vi "get All Data.vi"(0 "identifier":string, 1 "Board":u16, 2 "values":u16, 3 "id":u32, 4 "stats":dbl, 5 "advstats":cluster{}, 6 "spectra_size":u32, 7 "error in (no error)":errorcluster, 8 "data_number":u32) -> (18 "data_number out":u32, 20 "function return":bool, 22 "values out":u16, 23 "id out":u32, 24 "stats out":dbl, 25 "advstats out":cluster{}, 26 "spectra_size out":u32, 27 "error out":errorcluster)   [LabVIEW 2015, in "XGL_DPP.lvlib"]
doc: "EXTERN DECLSPEC bool CALL_CONV getAllData(const char * identifier,\n uint16_t Board,\n uint16_t * values,\n uint32_t * id,\n double* stats,\n uint64_t * advstats,\n uint32_t * spectra_size,\n uint32_t * data_number\n);"
uses:
  XGL_DPP.lvlib
  XGL_DPP.dll
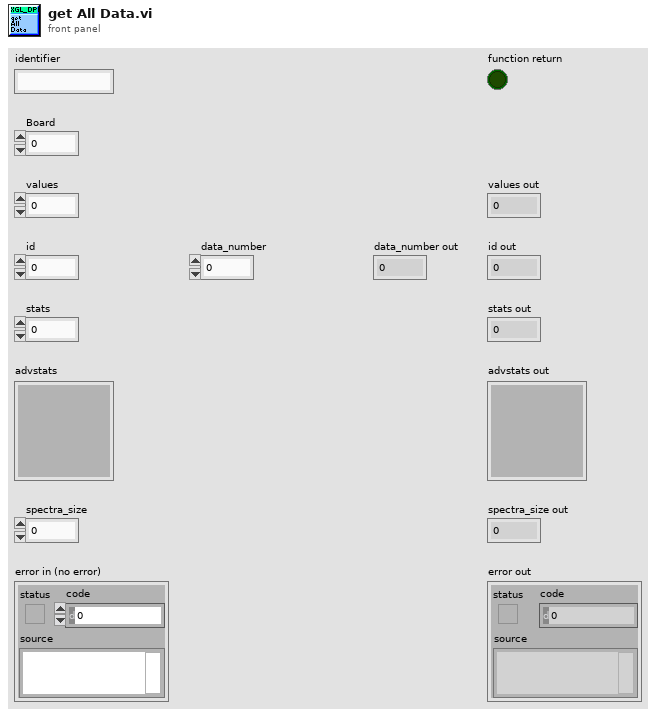
[diagram p1: front panel]
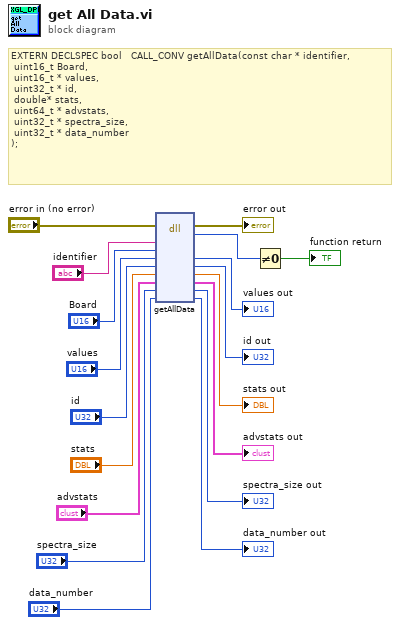
[diagram p0: block diagram]
diagram:
  # "EXTERN DECLSPEC bool   CALL_CONV getAllData(const char * identifier,\n\tuint16_t Board,\n\tuint16_t * values,\n\tuint32_t * id,\n\tdouble* stats,\n\tuint64_t * advstats,\n\tuint32_t * spectra_size,\n\tuint32_t * data_number\n);"
  n1 = dll-call lib="D:/Users/XRF/Desktop/Scanning Software_Demokritos_2015_v7/libs/Vis_2/XGL_DPP.*" fn="getAllData"(error in="error in (no error)", "identifier"="identifier", "Board"="Board", "values"="values", "id"="id", "stats"="stats", "advstats"="advstats", "spectra_size"="spectra_size", "data_number"="data_number") -> (error out=→"error out":errorcluster, w17:u8, "values"=→"values out":u16, "id"=→"id out":u32, "stats"=→"stats out":dbl, "advstats"=→"advstats out":cluster{}, "spectra_size"=→"spectra_size out":u32, "data_number"=→"data_number out":u32)  [unwired: 4 in, 1 out]
  n2 = Not Equal To 0?(x=w17) -> (x != 0?=→"function return":bool)
